vi "Loop Wrapper.vi"(9 "Error Queue":refnum<queue>, 10 "Event Actor Queue":refnum<queue>, 11 "Event Actor in":refnum<class "Event Actor.lvclass">) -> ()   [LabVIEW 2021, in "Event Actor.lvclass"]
uses:
  Event Actor.lvclass
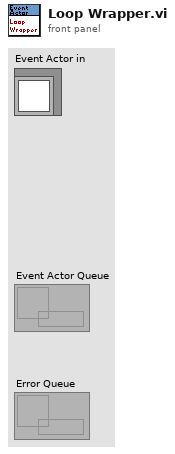
[diagram p1: front panel]
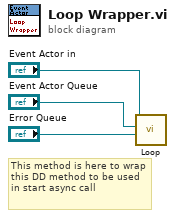
[diagram p0: block diagram]
diagram:
  # "This method is here to wrap this DD method to be used in start async call"
  n1 = call-dynamic "Loop.vi"("Error Queue"="Error Queue", "Event Actor Queue"="Event Actor Queue", "Event Actor in"="Event Actor in") -> ()  [unwired: 9 in]
